vi "TSCAN_CycliceWrite.vi"() -> ()   [LabVIEW 2019]
panel:
  in  "Cyclie":sgl
  in  "FIdxChn":i32(ring)=1 items=["CHN1", "CHN2", "CHN3", "CHN4", "CHN5", "CHN6", "CHN7", "CHN8", "CHN9", "CHN10", "CHN11", "CHN12", "CHN13", "CHN14", "CHN15", "CHN16", "CHN17", "CHN18", "CHN19", "CHN20", "CHN21", "CHN22", "CHN23", "CHN24", "CHN25", "CHN26", "CHN27", "CHN28", "CHN29", "CHN30", "CHN31", "CHN32"]
  in  "AIsExt":enum16{"STD", "EXT"}(ring)
  in  "ADataArray":u8[](array[numeric])
  in  "AID":u64 format="%x"
  out "路径输出":path
  in  "路径输入":path
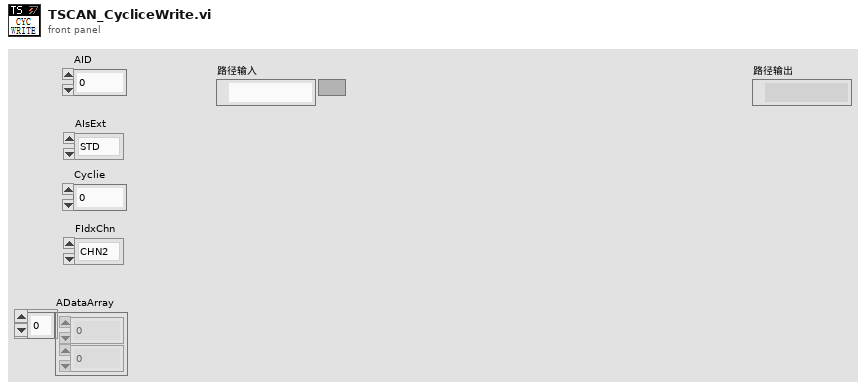
[diagram p1: front panel]
types:
  T1 = cluster{"FIdxChn":u8, "FProperties":u8, "FDLC":u8, "FReserved":u8, "FIdentifier":i32, "FTimeUS":u64, "Data0":u8, "Data1":u8, "Data2":u8, "Data3":u8, "Data4":u8, "Data5":u8, "Data6":u8, "Data7":u8}
  T2 = cluster{"istx":bool, "remoteframe":bool, "extframe":bool, "tbd1":bool, "tbd2":bool, "tbd3":bool, "tbd4":bool, "iserrorframe":bool}
  T3 = cluster{"AID":u32, "AIsExt":enum16{"STD", "EXT"}, "AIsRemote":enum16{"Data", "Remote"}, "ADLC":u8, "ADataArray":u8[], "FIdxChn":i32}
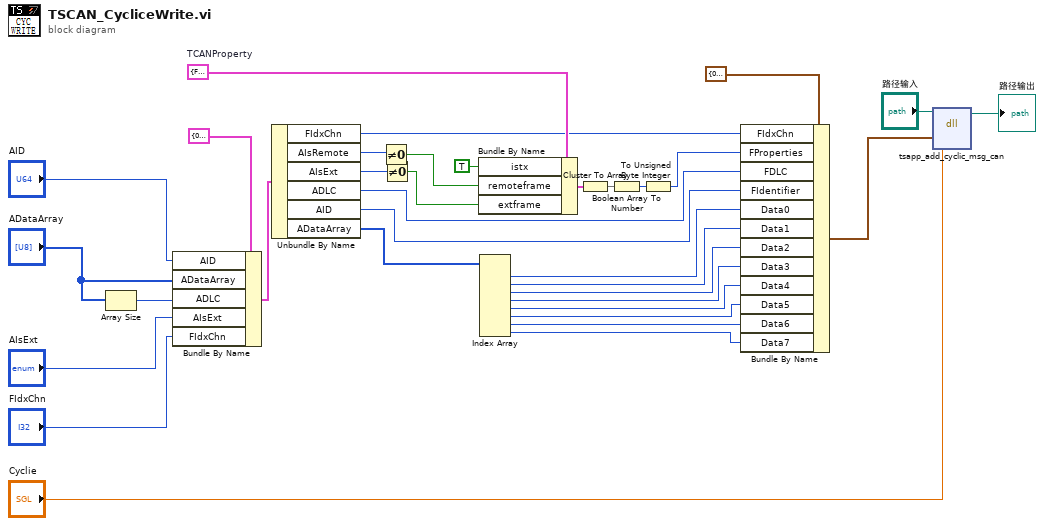
[diagram p0: block diagram]
diagram:
  w31 = T2 {"istx"=FALSE, "remoteframe"=FALSE, "extframe"=FALSE, "tbd1"=FALSE, "tbd2"=FALSE, "tbd3"=FALSE, "tbd4"=FALSE, "iserrorframe"=FALSE}  # TCANProperty
  n1 = Array Size(array="ADataArray") -> (size(s)=w8:i32)
  n2 = Bundle By Name(cluster=T3 {"AID"=0, "AIsExt"=enum."STD", "AIsRemote"=enum."Data", "ADLC"=0, "ADataArray"=[], "FIdxChn"=1} ("数据帧信息"), "AID"="AID", "ADataArray"="ADataArray", "ADLC"=w8, "AIsExt"="AIsExt", "FIdxChn"="FIdxChn") -> (w7:T3)
  n3 = Unbundle By Name(w7) -> ("FIdxChn"=w27:i32, "AIsRemote"=w24:enum16{"Data", "Remote"}, "AIsExt"=w22:enum16{"STD", "EXT"}, "ADLC"=w20:u8, "AID"=w19:u32, "ADataArray"=w18:u8[])
  n4 = Not Equal To 0?(x=w24) -> (x != 0?=w23:bool)
  n5 = Not Equal To 0?(x=w22) -> (x != 0?=w21:bool)
  n6 = Bundle By Name(cluster=w31, "istx"=TRUE, "remoteframe"=w23, "extframe"=w21) -> (w26:T2)
  n7 = Index Array(array=w18) -> (element #1=w17:u8, element #2=w16:u8, element #3=w15:u8, element #4=w14:u8, element #5=w13:u8, element #6=w12:u8, element #7=w11:u8, element #8=w10:u8)  [unwired: 8 in]
  n8 = Cluster To Array(cluster=w26) -> (array=w29:bool[])
  n9 = Boolean Array To Number(Boolean array=w29) -> (number=w28:u32)
  n10 = To Unsigned Byte Integer(number=w28) -> (unsigned 8bit integer=w25:u8)
  n11 = Bundle By Name(cluster=T1 {"FIdxChn"=0, "FProperties"=0, "FDLC"=0, "FReserved"=0, "FIdentifier"=0, "FTimeUS"=0, "Data0"=0, "Data1"=0, "Data2"=0, "Data3"=0, "Data4"=0, "Data5"=0, "Data6"=0, "Data7"=0} ("SendMsgInfo"), "FIdxChn"=w27, "FProperties"=w25, "FDLC"=w20, "FIdentifier"=w19, "Data0"=w17, "Data1"=w16, "Data2"=w15, "Data3"=w14, "Data4"=w13, "Data5"=w12, "Data6"=w11, "Data7"=w10) -> (w4:T1)
  n12 = dll-call lib="PTH2Zabs CUsers\nAdministratorDesktop海卓电堆系统程序\nTS_CAN_ModTSMaster.dll" fn="tsapp_add_cyclic_msg_can"(path in="路径输入", "ACAN"=w4, "Cyclie"="Cyclie") -> (path out=→"路径输出":path)  [unwired: 5 in, 1 out]
